vi "Unregister (async).vi"(8 "error in (no error)":errorcluster, 9 "Endpoint URI":string, 11 "WAMP Client in":refnum<class "WAMP Client.lvclass">) -> (0 "error out":errorcluster, 1 "Sucess or error":refnum<user-event>, 3 "WAMP Client out":refnum<class "WAMP Client.lvclass">)   [LabVIEW 2020, in "wamplv.lvlib" / "WAMP Client.lvclass"]
uses:
  WAMP Client.lvclass
  TypeDef/Success or error.ctl
  TypeDefs/Combined error.ctl
  TypeDefs/WAMP error.ctl
  TypeDef/Internal Message Type.ctl
  TypeDef/Unregister request.ctl
  WAMP Client.lvclass/WAMP Client.ctl
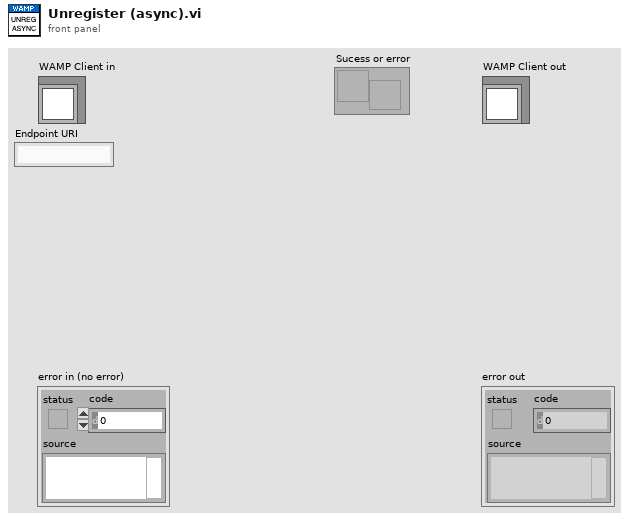
[diagram p1: front panel]
types:
  T1 = typedef "wamplv.lvlib/WAMP Client.lvclass/Unregister request.ctl" = cluster{"URI":string, "Unregister user event":refnum<user-event>}
  T2 = typedef "wamplv.lvlib/WAMP Client.lvclass/Success or error.ctl" = cluster{"Success?":bool, "URI":string, "Combined Error":T3}
  T3 = typedef "wamplv.lvlib/WAMP Client.lvclass/Combined error.ctl" = cluster{"Error?":bool, "WAMP Error":T4, "Error":errorcluster}
  T4 = typedef "wamplv.lvlib/WAMP Client.lvclass/WAMP error.ctl" = cluster{"Details":string, "ArgumentKw Payload":string, "Error?":bool, "Error URI":string, "Arguments Payload":string[]}
  T5 = typedef "wamplv.lvlib/WAMP Client.lvclass/Internal Message Type.ctl" = enum16{"Subscribe", "Handle Subscribed", "Handle Event", "Unsubscribe", "Handle Unsubscribed", "Publish", "Handled Published", "Goodbye", "Handle Goodbye", "Call", "Handle Result", "Register", "Handle Registered", "Unregister", "Handle Unregistered", "Handle Invocation", "Yield", "Error"}
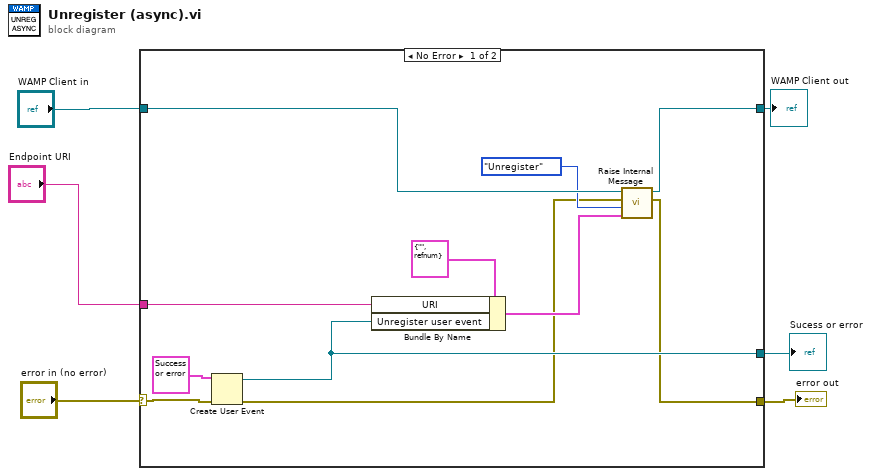
[diagram p0: block diagram]
diagram:
  n1 = case shown="No Error" "error in (no error)" {
    selector: "error in (no error)" -> [w10 w19]
    tunnel: [w8 w19] -> w5
    tunnel: [w7 w18] -> w3
    tunnel: "WAMP Client in" -> [w17 w18]
    tunnel: [w14 _] -> w1
    tunnel: "Endpoint URI" -> [w15 _]
    frame No Error {
      n2 = Create User Event(user event datatype=T2 {"Success?"=FALSE, "URI"="", "Combined Error"={"Error?"=FALSE, "WAMP Error"={"Details"="{}", "ArgumentKw Payload"="{}", "Error?"=FALSE, "Error URI"="", "Arguments Payload"=[]}, "Error"={"status"=FALSE, "code"=0, "source"=""}}} ("Sucess or error"), error in=w10) -> (user event=w14:refnum<user-event>, error out=w9:errorcluster)
      n3 = Bundle By Name(cluster=T1 {"URI"="", "Unregister user event"=refnum} ("Unregister Request"), "URI"=w15, "Unregister user event"=w14) -> (w16:T1)
      n4 = call-dynamic "Raise Internal Message.vi"("Variant"=w16, "Internal Message Type"=Internal_Message_Type."Unregister", "error in (no error)"=w9, "WAMP Client in"=w17) -> ("error out"=w8:errorcluster, "WAMP Client out"=w7:refnum<class "WAMP Client.lvclass">)  [unwired: 6 in]
    }
    frame Error {
    }
  }
  "error out" <- w5
  "WAMP Client out" <- w3
  "Sucess or error" <- w1
